vi "GCMPlugin_IsSupportingItem.vi"(8 "error in (no error)":errorcluster, 9 "VI Reference":refnum<vi>, 10 "ProjectItem Refnum":refnum<vi>, 11 "TemplatePlugin in":refnum<class "EXESpecEditor.lvclass">) -> (0 "error out":errorcluster, 2 "IsSupportingItem":bool, 3 "TemplatePlugin out":refnum<class "EXESpecEditor.lvclass">)   [LabVIEW 2014, in "BuildSpecEditor.lvlib" / "EXESpecEditor.lvclass"]
uses:
  EXESpecEditor.lvclass
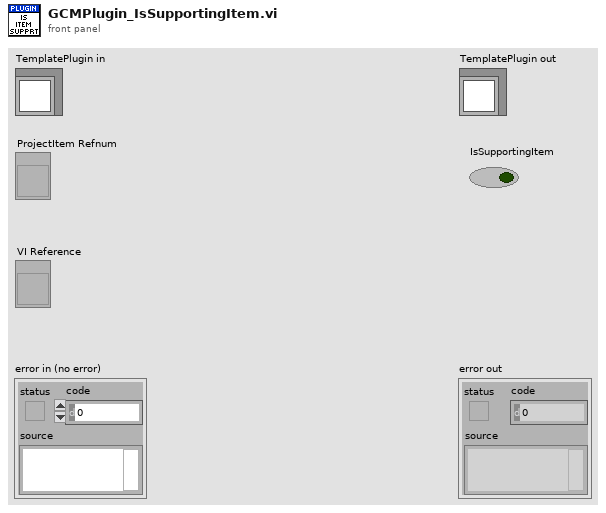
[diagram p1: front panel]
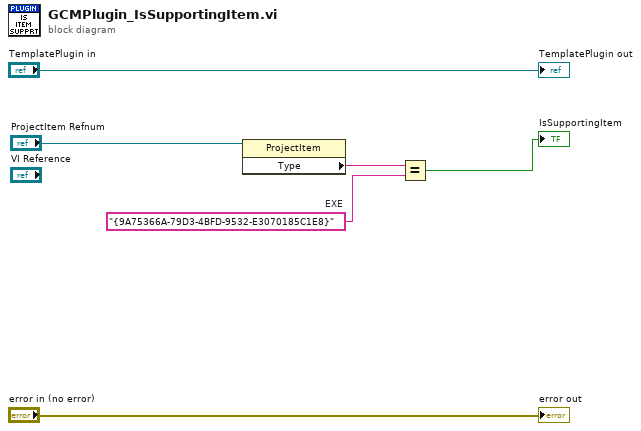
[diagram p0: block diagram]
diagram:
  w3 = "{9A75366A-79D3-4BFD-9532-E3070185C1E8}"  # EXE
  n1 = property class="ProjectItem"(reference="ProjectItem Refnum") -> ("Type"=w2:string)  [unwired: 1 in, 2 out]
  n2 = Equal?(x=w2, y=w3) -> (x = y?=→"IsSupportingItem":bool)
  "error out" <- "error in (no error)"
  "TemplatePlugin out" <- "TemplatePlugin in"
